vi "Set Sample Rate.vi"(8 "error in (no error)":errorcluster, 10 "Sample Rate":i32, 11 "Graph Manager in":refnum<class "Graph Manager.lvclass">) -> (0 "error out":errorcluster, 3 "Graph Manager out":refnum<class "Graph Manager.lvclass">)   [LabVIEW 2016, in "Graph Manager.lvclass"]
uses:
  Graph Manager.lvclass
  Graph Manager.lvclass/Graph Manager.ctl
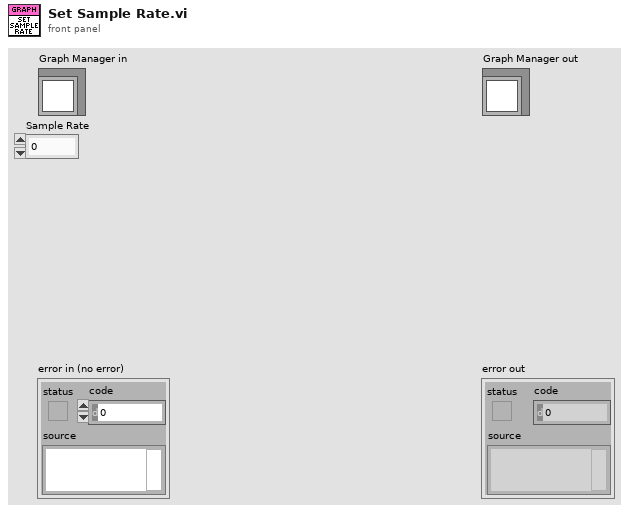
[diagram p1: front panel]
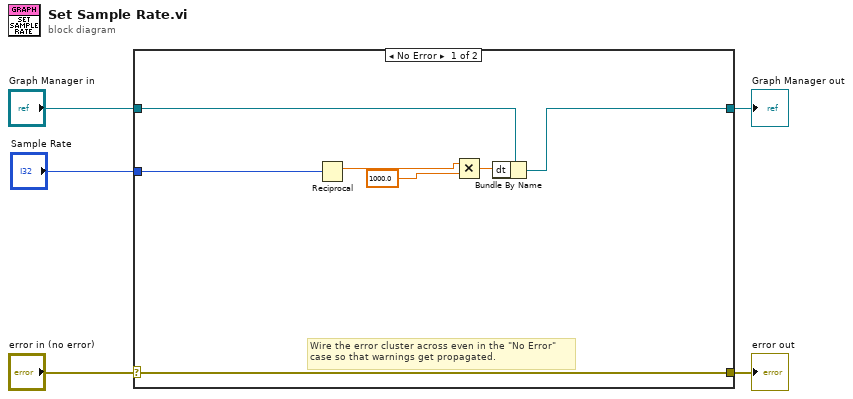
[diagram p0: block diagram]
diagram:
  n1 = case shown="No Error" "error in (no error)" {
    selector: "error in (no error)" -> [w12 w14]
    tunnel: [w12 w14] -> w4
    tunnel: [w10 w13] -> w2
    tunnel: "Graph Manager in" -> [w11 w13]
    tunnel: "Sample Rate" -> [w9 _]
    frame No Error {
      # "Wire the error cluster across even in the \"No Error\"\ncase so that warnings get propagated."
      n2 = Reciprocal(x=w9) -> (1/x=w8:dbl)
      n3 = Multiply(x=w8, y=1000.0) -> (x*y=w6:dbl)
      n4 = Bundle By Name(cluster=w11, "dt"=w6) -> (w10:refnum<class "Graph Manager.lvclass">)
    }
    frame Error {
    }
  }
  "error out" <- w4
  "Graph Manager out" <- w2
